vi "ViewStringNotepad.vi"(11 "Input":string) -> ()   [LabVIEW 2016]
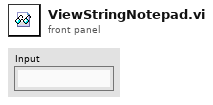
[diagram p1: front panel]
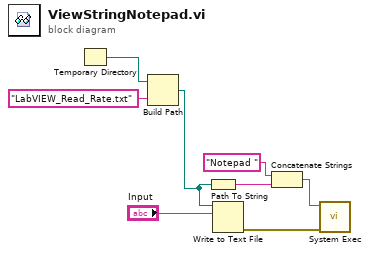
[diagram p0: block diagram]
diagram:
  n1 = Temporary Directory() -> (w3:path)
  n2 = Build Path(base path=w3, name or relative path="LabVIEW_Read_Rate.txt") -> (appended path=w2:path)
  n3 = Path To String(path=w2) -> (string=w8:string)
  n4 = Write to Text File(file (use dialog)=w2, text="Input") -> (error out=w5:errorcluster)  [unwired: 2 in, 2 out]
  n5 = Concatenate Strings("Notepad " ("string"), w8) -> (w6:string)
  n6 = call <vilib>:"System Exec.vi"("error in (no error)"=w5, "command line"=w6) -> ()  [unwired: 6 in, 4 out]
